vi "SNED_FLOAT_T_CHANNEL_V_S.vi"(1 "数据":dbl, 2 "电压or位移":string, 3 "通道":dbl, 4 "T":string) -> (0 "处理之后的数据":string)   [LabVIEW 2014]
panel:
  out "校验之后的数据":u8
  out "第一个校验数据":u8
  out "String 2":string
  out "4":u8
  out "3":u8
  out "2":u8
  out "1":u8
  out "String":string
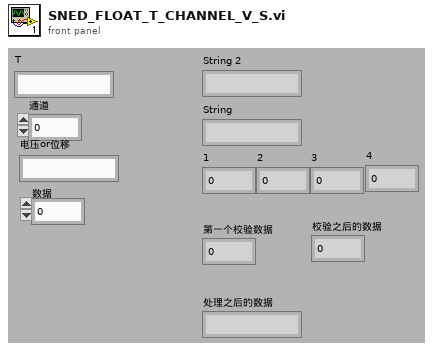
[diagram p1: front panel]
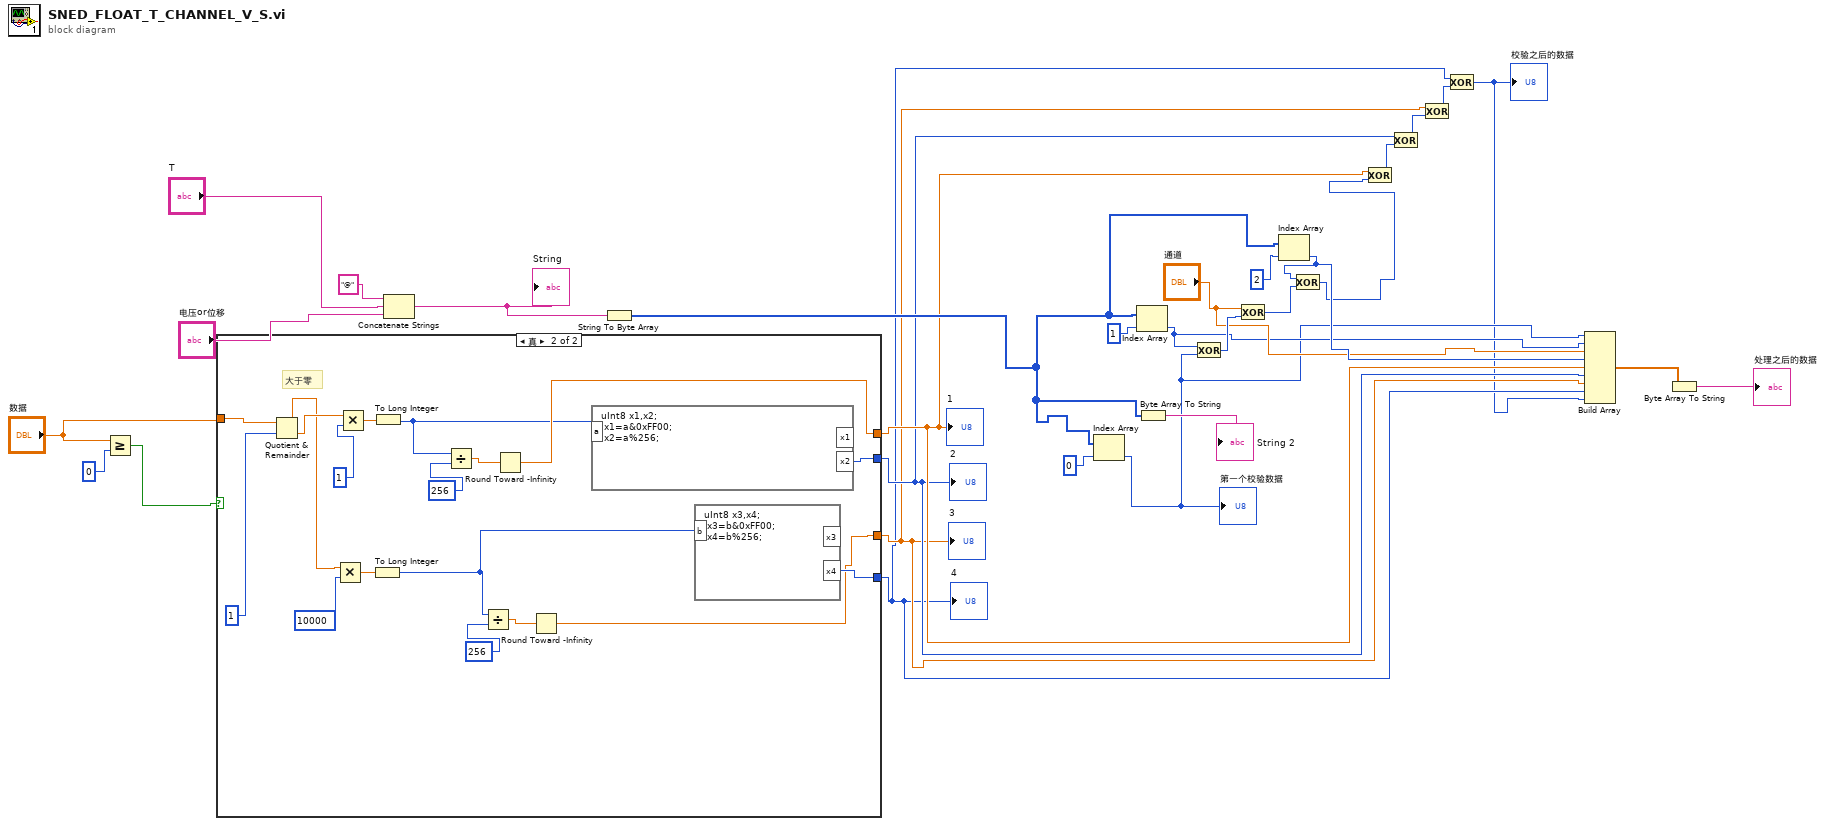
[diagram p0: block diagram]
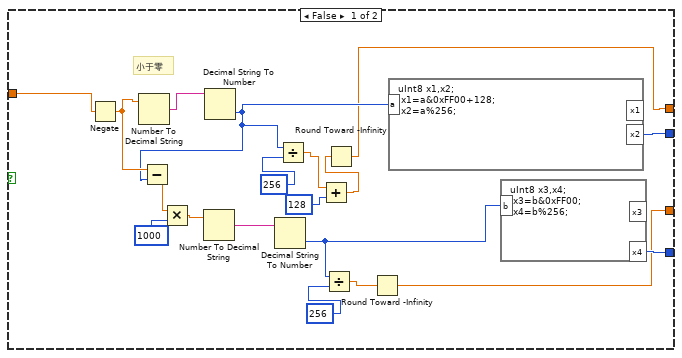
[diagram p2: hidden frame]
diagram:
  n1 = Greater Or Equal?(x="数据", y=0) -> (x >= y?=w1:bool)
  n2 = case shown="真" w1 {
    tunnel: "数据" -> [w44 w58]
    tunnel: [w38 w60] -> w8
    tunnel: [w42 w66] -> w7
    tunnel: [w33 w59] -> w6
    tunnel: [w41 w65] -> w5
    frame False {
      # "小于零"
      n3 = Negate(x=w44) -> (-x=w43:dbl)
      n4 = Number To Decimal String(number=w43) -> (decimal integer string=w45:string)  [unwired: 1 out]
      n5 = Decimal String To Number(string=w45) -> (number=w39:i32)  [unwired: 3 out]
      n6 = Subtract(x=w43, y=w39) -> (x-y=w48:dbl)
      n7 = Multiply(x=w48, y=1000) -> (x*y=w46:dbl)
      n8 = Number To Decimal String(number=w46) -> (decimal integer string=w35:string)  [unwired: 1 out]
      n9 = Decimal String To Number(string=w35) -> (number=w34:i32)  [unwired: 3 out]
      n10 = Divide(x=w39, y=256) -> (x/y=w32:dbl)
      n11 = Add(x=w32, y=128) -> (x+y=w30:dbl)
      n12 = Divide(x=w34, y=256) -> (x/y=w37:dbl)
      n13 = Round Toward -Infinity(1:w30) -> (0:w38:dbl)
      n14 = Round Toward -Infinity(1:w37) -> (0:w33:dbl)
      n15 = formula code="uInt8 x1,x2;\n x1=a&0xFF00+128;\n x2=a%256;"("a"=w39) -> ("x2"=w42:u8)  [unwired: 1 out]
      n16 = formula code="uInt8 x3,x4;\n x3=b&0xFF00;\n x4=b%256;"("b"=w34) -> ("x4"=w41:u8)  [unwired: 1 out]
    }
    frame True {
      # "大于零"
      n17 = Quotient & Remainder(x=w58, y=1) -> (x-y*floor(x/y)=w49:dbl, floor(x/y)=w50:dbl)
      n18 = Multiply(x=w49, y=10000) -> (x*y=w54:dbl)
      n19 = Multiply(x=w50, y=1) -> (x*y=w52:dbl)
      n20 = To Long Integer(number=w54) -> (32bit integer=w51:i32)
      n21 = To Long Integer(number=w52) -> (32bit integer=w53:i32)
      n22 = Divide(x=w53, y=256) -> (x/y=w62:dbl)
      n23 = Divide(x=w51, y=256) -> (x/y=w64:dbl)
      n24 = Round Toward -Infinity(1:w62) -> (0:w60:dbl)
      n25 = Round Toward -Infinity(1:w64) -> (0:w59:dbl)
      n26 = formula code="uInt8 x1,x2;\n x1=a&0xFF00;\n x2=a%256;"("a"=w53) -> ("x2"=w66:u8)  [unwired: 1 out]
      n27 = formula code="uInt8 x3,x4;\n x3=b&0xFF00;\n x4=b%256;"("b"=w51) -> ("x4"=w65:u8)  [unwired: 1 out]
    }
  }
  "1" <- w8
  "2" <- w7
  "3" <- w6
  "4" <- w5
  n28 = Concatenate Strings("@", "T", "电压or位移") -> (w28:string)
  "String" <- w28
  n29 = String To Byte Array(string=w28) -> (unsigned byte array=w15:u8[])
  n30 = Index Array(array=w15, index=0) -> (element=w10:u8)
  "第一个校验数据" <- w10
  n31 = Index Array(array=w15, index=1) -> (element=w11:u8)
  n32 = Byte Array To String(unsigned byte array=w15) -> (string=→"String 2":string)
  n33 = Exclusive Or(1:w10, 2:w11) -> (0:w17:u8)
  n34 = Exclusive Or(1:w17, 2:"通道") -> (0:w14:i32)
  n35 = Index Array(array=w15, index=2) -> (element=w13:u8)
  n36 = Exclusive Or(1:w14, 2:w13) -> (0:w9:i32)
  n37 = Exclusive Or(1:w9, 2:w8) -> (0:w24:i32)
  n38 = Exclusive Or(1:w24, 2:w7) -> (0:w23:i32)
  n39 = Exclusive Or(1:w23, 2:w6) -> (0:w22:i32)
  n40 = Exclusive Or(1:w22, 2:w5) -> (0:w4:i32)
  "校验之后的数据" <- w4
  n41 = Build Array(w10, w11, "通道", w13, w8, w7, w6, w5, w4) -> (w21:dbl[])
  n42 = Byte Array To String(unsigned byte array=w21) -> (string=→"处理之后的数据":string)
